vi "terminate.vi"(8 "error in (no error)":errorcluster, 11 "GenericPlugin in":refnum<class "GenericToplevelComponent.lvclass">) -> (0 "error out":errorcluster, 3 "GenericPlugin out":refnum<class "GenericToplevelComponent.lvclass">)   [LabVIEW 2010, in "GenericToplevelComponent.lvclass"]
doc: "The dynamic dispatch version of this VI terminates the plug-in object by releasing all of its resources."
uses:
  GenericToplevelComponent.lvclass
  GenericComponent/GenericComponent/GenericComponent.lvclass
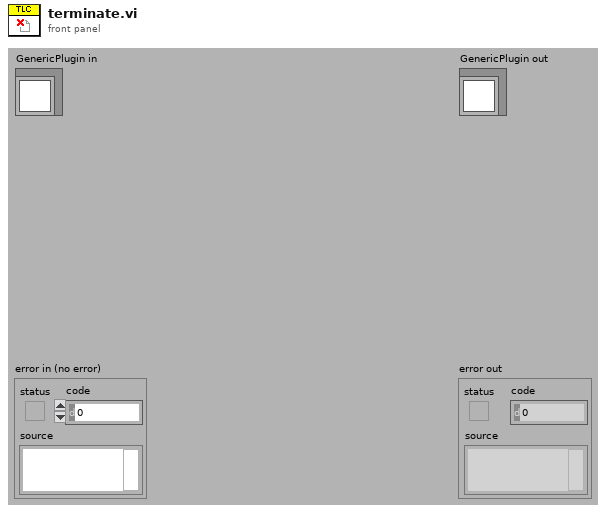
[diagram p1: front panel]
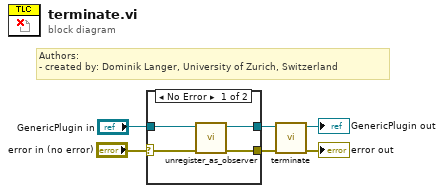
[diagram p0: block diagram]
diagram:
  # "Authors: \n- created by: Dominik Langer, University of Zurich, Switzerland"
  n1 = case shown="No Error" "error in (no error)" {
    selector: "error in (no error)" -> [w7 w11]
    tunnel: [w10 w11] -> w4
    tunnel: "GenericPlugin in" -> [w9 w12]
    tunnel: [w8 w12] -> w2
    frame No Error {
      n2 = call-dynamic "unregister_as_observer.vi"("error in (no error)"=w7, "GenericToplevelComponent in"=w9) -> ("error out"=w10:errorcluster, "GenericToplevelComponent out"=w8:refnum<class "GenericToplevelComponent.lvclass">)  [unwired: 8 in]
    }
    frame Error {
    }
  }
  n3 = call-parent "terminate.vi"("error in (no error)"=w4, "GenericPlugin in"=w2) -> ("error out"=→"error out":errorcluster, "GenericPlugin out"=→"GenericPlugin out":refnum<class "GenericToplevelComponent.lvclass">)  [unwired: 8 in]
